vi "CurveDrive.vi"(8 "error in":errorcluster, 11 "Joystick":dbl format="%#_13g") -> (0 "error out":errorcluster, 3 "Throttle":dbl)   [LabVIEW 2015]
panel:
  in  "exponent":dbl=1.8 format="%#_13g"
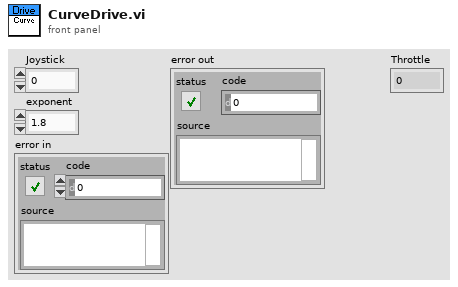
[diagram p1: front panel]
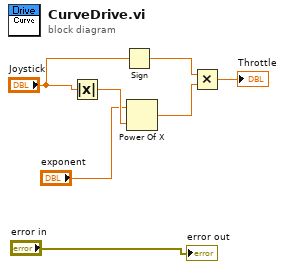
[diagram p0: block diagram]
diagram:
  n1 = Absolute Value(x="Joystick") -> (abs(x)=w5:dbl)
  n2 = Sign(1:"Joystick") -> (0:w7:dbl)
  n3 = Power Of X(1:w5, 2:"exponent") -> (0:w3:dbl)
  n4 = Multiply(x=w7, y=w3) -> (x*y=→"Throttle":dbl)
  "error out" <- "error in"
